vi "APC_PC_UI_System.vi"() -> ()   [LabVIEW 2020]
uses:
  controls/APC_PIDcontrolSettings.ctl
  <vilib>/Modbus/master/Create Master Instance (TCP).vi
  <vilib>/Modbus/master/Modbus Master.lvclass
panel:
  in  "Tab Control 2":enum32{"System view", "MTR interface", "Other"}(tab)
  out "WF-PT-012avg":dbl caption="bar" format="%#.2f"
  out "NG_CL_inner":bool
  in  "Ar_direct":bool
  in  "Ar_CL_inner":bool
  in  "AR-FT-001-REF":dbl caption="kg/h" format="%#.2f"
  in  "O2_direct":bool
  in  "Tcoolant_direct":bool
  in  "Toil_direct":bool
  in  "Texh_direct":bool
  out "SW-TT-009":dbl caption="ºC" format="%#.1f"
  out "NGDI-TT-001":dbl caption="ºC" format="%#.1f"
  out "NGDI-PT-001":dbl caption="bar" format="%#.2f"
  out "NG-TT-001":dbl caption="ºC" format="%#.1f"
  out "NG-PT-001":dbl caption="bar" format="%#.2f"
  in  "O2_FF_NG":bool
  out "Emergency shutdown":bool
  out "Pre-operation":bool
  out "Operation":bool
  out "Start":bool
  out "Idle":bool
  out "Shutdown":bool
  out "MTR errors":bool[](array[boolean])
  out "HB":bool
  out "Control from LV":bool
  in  "MTR_CO2out_CL":bool
  in  "IMEP-REF":dbl caption="l" format="%#.2f"
  out "NG_CL_outer_IMEP":bool caption="NG_CL_outer"
  out "NG_CL_outer_Nm":bool caption="NG_CL_outer"
  in  "TORQUE-REF":dbl caption="l" format="%#.2f"
  out "9056":bool
  out "9049":bool
  out "TORQUE":dbl caption="Nm" format="%#.2f"
  in  "Toil_CL_outer":bool
  out "Stand-by":bool
  out "Motoring":bool
  out "Firing":bool
  out "Idling":bool
  out "Emergency":bool
  in  "Tcoolant_CL":bool
  in  "Toil_CL_inner":bool
  out "Pmax-6":dbl caption="bar" format="%#.2f"
  out "Pmax-5":dbl caption="bar" format="%#.2f"
  out "Pmax-4":dbl caption="bar" format="%#.2f"
  out "Pmax-3":dbl caption="bar" format="%#.2f"
  out "Pmax-2":dbl caption="bar" format="%#.2f"
  out "Pmax-1":dbl caption="bar" format="%#.2f"
  out "IMEP-6":dbl caption="bar" format="%#.2f"
  out "IMEP-5":dbl caption="bar" format="%#.2f"
  out "IMEP-4":dbl caption="bar" format="%#.2f"
  out "IMEP-3":dbl caption="bar" format="%#.2f"
  out "IMEP-2":dbl caption="bar" format="%#.2f"
  out "IMEP-1":dbl caption="bar" format="%#.2f"
  out "PC-TT-006":dbl caption="ºC" format="%#.1f"
  out "PC-TT-005":dbl caption="ºC" format="%#.1f"
  out "PC-TT-004":dbl caption="ºC" format="%#.1f"
  out "PC-TT-003":dbl caption="ºC" format="%#.1f"
  out "PC-TT-002":dbl caption="ºC" format="%#.1f"
  out "PC-TT-001":dbl caption="ºC" format="%#.1f"
  out "EO-PT-001":dbl caption="bar" format="%#.2f"
  out "EO-TT-002":dbl caption="ºC" format="%#.1f"
  out "RPM":dbl caption="rpm" format="%#.1f"
  in  "EMERGENCY STOP":bool
  in  "Clear warning":bool
  in  "Exhaust vent":bool
  in  "Cross vent":bool
  in  "Intake vent":bool
  in  "O2":bool
  in  "Ar":bool
  in  "NG":bool
  in  "MTR_BackPressure_CL":bool
  in  "Texh_CL_outer":bool
  in  "Texh_CL_inner":bool
  in  "MTR_BackFlow_CL":bool
  in  "CO2_CL_inner":bool
  in  "CO2_CL_outer":bool
  out "NG_CL_outer_lambda":bool caption="NG_CL_outer"
  in  "O2_CL":bool
  in  "AR_CL_outer":bool
  out "AT201_CO2Conc":dbl caption="[% CO2]" format="%#.2f"
  in  "AIC201_CO2_ConcTarget":dbl caption="[% CO2]" format="%#.2f"
  in  "PV300_VlvPosTarget_pc":dbl caption="%" format="%#.2f"
  out "PV300_VlvPos_pc_fb":dbl caption="%" format="%#.2f"
  out "PT300_Pressure_kPa":dbl caption="bar" format="%#.2f"
  in  "PV300_PressTarget_kPa":dbl caption="bar" format="%#.2f"
  in  "WF-TT-004-REF":dbl caption="ºC"
  out "AT103_CO2Conc":dbl caption="[% CO2]" format="%#.2f"
  in  "AIC103_CO2_ConcTarget":dbl caption="[% CO2]" format="%#.2f"
  in  "PV103_VlvPosTarget_pc":dbl caption="%" format="%#.2f"
  out "PV103_VlvPos_pc_fb":dbl caption="%" format="%#.2f"
  out "PT103_Pressure_kPa":dbl caption="bar" format="%#.2f"
  in  "PV103_PressTarget_kPa":dbl caption="bar" format="%#.2f"
  in  "FV301_VlvPosTarget_pc":dbl caption="%" format="%#.2f"
  out "FV301_VlvPos_pc_fb":dbl caption="%" format="%#.2f"
  in  "FV301_FlowTarget_kgh":dbl caption="kg/h" format="%#.2f"
  in  "SW-FC-004-REF":dbl caption="%" format="%#.2f"
  out "SW-FC-004":dbl caption="%" format="%#.2f"
  in  "SW-FT-002-REF":dbl caption="kg/h" format="%#.2f"
  in  "SW-FC-008-REF":dbl caption="%" format="%#.2f"
  out "SW-FC-009":dbl caption="%" format="%#.2f"
  in  "EO-TT-001-REF":dbl caption="ºC"
  out "EO-TT-001":dbl caption="ºC" format="%#.1f"
  in  "SW-FT-004-REF":dbl caption="kg/h" format="%#.2f"
  out "WF-TT-007":dbl caption="ºC" format="%#.1f"
  out "WF-PT-016":dbl caption="bar" format="%#.2f"
  out "WF-PT-014":dbl caption="bar" format="%#.2f"
  out "WF-TT-003":dbl caption="ºC" format="%#.1f"
  in  "NG-FC-001-REF":dbl caption="kg/h" format="%#.2f"
  out "NG-FC-001":dbl caption="kg/h" format="%#.2f"
  out "ExhVent":bool
  out "O2":bool
  out "Ar":bool
  out "NG":bool
  out "CrossVent":bool
  out "IntVent":bool
  in  "EC-FC-001-REF":dbl caption="%"
  out "EC-FC-001":dbl caption="%"
  in  "EC-TT-001-REF":dbl caption="ºC"
  in  "WF-OA-002-REF":dbl caption="l" format="%#.2f"
  in  "AR-PC-002-REF":dbl caption="bar" format="%#.2f"
  in  "O2-FC-001-REF":dbl caption="kg/h" format="%#.2f"
  in  "WF-OA-001-REF":dbl caption="[% O2]" format="%#.2f"
  out "WF-TT-004":dbl caption="ºC" format="%#.1f"
  out "PT104_Pressure_kPa":dbl caption="bar" format="%#.2f"
  out "PT106_Pressure_kPa":dbl caption="bar" format="%#.2f"
  out "C101_CompSpeed_rpm":dbl caption="rpm"
  out "SW-TT-002":dbl caption="ºC" format="%#.1f"
  out "SW-TT-001":dbl caption="ºC" format="%#.1f"
  out "SW-TT-003":dbl caption="ºC" format="%#.1f"
  out "SW-TT-004":dbl caption="ºC" format="%#.1f"
  out "SW-TT-008":dbl caption="ºC" format="%#.1f"
  out "SW-TT-007":dbl caption="ºC" format="%#.1f"
  out "SW-TT-005":dbl caption="ºC" format="%#.1f"
  out "SW-TT-006":dbl caption="ºC" format="%#.1f"
  out "EC-TT-001":dbl caption="ºC" format="%#.1f"
  out "EC-TT-002":dbl caption="ºC" format="%#.1f"
  out "WF-OA-001":dbl caption="[% O2]" format="%#.2f"
  out "WF-PT-005avg":dbl caption="bar" format="%#.2f"
  out "WF-PT-004":dbl caption="bar" format="%#.2f"
  out "WF-OA-002":dbl caption="l" format="%#.2f"
  out "WF-TT-002":dbl caption="ºC" format="%#.1f"
  out "O2-TT-001":dbl caption="ºC" format="%#.1f"
  out "O2-PT-001":dbl caption="bar" format="%#.2f"
  out "AR-TT-001":dbl caption="ºC" format="%#.1f"
  out "AR-PT-001":dbl caption="bar" format="%#.2f"
  out "WF-TT-001":dbl caption="ºC" format="%#.1f"
  out "WF-PT-001":dbl caption="bar" format="%#.2f"
  out "FT301_Flow_kgh":dbl caption="kg/h" format="%#.2f"
  out "SW-FT-002":dbl caption="kg/h" format="%#.2f"
  out "SW-FT-003":dbl caption="kg/h" format="%#.2f"
  out "SW-FT-001":dbl caption="kg/h" format="%#.2f"
  out "SW-FT-004":dbl caption="kg/h" format="%#.2f"
  out "O2-FC-001":dbl caption="kg/h" format="%#.2f"
  out "NG-FT-001":dbl caption="kg/h" format="%#.2f"
  out "AR-FT-001":dbl caption="kg/h" format="%#.2f"
  out "NGDI-FT-001":dbl caption="kg/h" format="%#.1f"
  in  "WF-PT-003-REF":dbl caption="bar" format="%#.2f"
  out "NOx":dbl caption="[ppm NOx]" format="%#.1f"
  in  "port (502)":u16=502
  in  "Slave address":string="172.22.11.1"
  out "error out":errorcluster
  in  "min 2":sgl[](array[numeric])=[0.0, 0.0, 0.0, 0.0, 0.0, 0.0, 0.0, 0.0, 0.0, 0.0, 0.0, 0.0, 0.0, 0.0, 0.0, 0.0, 0.0, 0.0, 0.0]
  in  "max 2":sgl[](array[numeric])=[100.0, 100.0, 300.0, 300.0, 100.0, 100.0, 100.0, 100.0, 500.0, 500.0, 100.0, 100.0, 200.0, 200.0, 100.0, 100.0, 40000.0, 300.0, 600.0]
  out "MTR modbus floats":sgl[](array[numeric])
  in  "max":sgl[](array[numeric])=[100.0, 300.0, 100.0, 100.0, 500.0, 100.0, 200.0, 100.0]
  in  "min":sgl[](array[numeric])=[0.0, 0.0, 0.0, 0.0, 0.0, 0.0, 0.0, 0.0]
  in  "Send2MTRuint16":u16[](array[numeric])=[0, 0, 0]
  in  "Send2MTRfloats":sgl[](array[numeric])=[0.0, 0.0, 0.0, 0.0, 0.0, 0.0, 0.0, 0.0]
  out "MTR modbus u16":u16[](array[numeric])
  out "Texh control mode":u8
  out "PV300_Ctrl_Mode":u16
  out "FV301_Ctrl_Mode":u16
  out "NG control mode":u8
  out "Ar control mode":u8
  out "O2 control mode":u8
  out "Tcoolant control  mode":u8
  out "PV103_Ctrl_Mode":u16
  out "OverrideFromMain":bool
  out "Toil control mode":u8
  # "monarch APC v0.1"
  # "NG"
  # "T exh"
  # "IMEP"
  # "peak P"
  # "AR"
  # "NG FF"
  # "coolant"
  # "O2"
  # "oil"
  # "RT HB"
  # "Main switches"
  # "Membrane warnings"
  # "0 - M101 inlet T HH\n1 - M101 inlet p HH\n2 - S101 level HH\n3 - C101 inlet p LL\n4 - C101 inlet p HH\n5 - C101 outlet p HH\n6 - C101 outlet T HH\n7 - Oil p LL\n8 - Oil T HH\n9 - S102 level HH\n10 - M102 inlet T HH\n11 - CO2 exhaust T LL"
  # "M101"
  # "S102"
  # "C101"
  # "S101"
  # "drain"
  # "Membrane state"
  # "CO2"
  # "M102"
  # "AIC103_CO2_ConcTarget\nPV103_PressTarget_kPa\nPV103_VlvPosTarget_pc\nAIC201_CO2_ConcTarget\nFV301_FlowTarget_kgh\nFV301_VlvPosTarget_pc\nPV300_PressTarget_kPa\nPV300_VlvPosTarget_pc"
  # "PV103_Ctrl_Mode\nFV301_Ctrl_Mode\nPV300_Ctrl_Mode"
  # "AIC103_CO2_ConcTarget_ack\nAT103_CO2Conc\nPV103_PressTarget_kPa_ack\nPT103_Pressure_kPa\nPV103_VlvPosTarget_pc_ack\nPV103_VlvPos_pc_fb\nAIC201_CO2_ConcTarget_ack\nAT201_CO2Conc\nFV301_FlowTarget_kgh_ack\nFT301_Flow_kgh\nFV301_VlvPosTarget_pc_ack\nFV301_VlvPos_pc_fb\nPV300_PressTarget_kPa_ack\nPT300_Pressure_kPa\nPV300_VlvPosTarget_pc_ack\nPV300_VlvPos_pc_fb\nC101_CompSpeed_rpm\nPT104_Pressure_kPa\nPT106_Pressure_kPa"
  # "PLC_Manual_Control\nMTR_State\nMTR_HeartBeat\nPV103_Ctrl_Mode_act\nFV301_Ctrl_Mode_act\nPV300_Ctrl_Mode_act\nMTR_Diagnostic_Status"
  # "0 - Undefined\n1 - Idle\n2 - Start\n3 - Pre-Operation\n4 - Operation\n5 - ShutDown\n6 - Emergency ShutDown (ESD triggered!)"
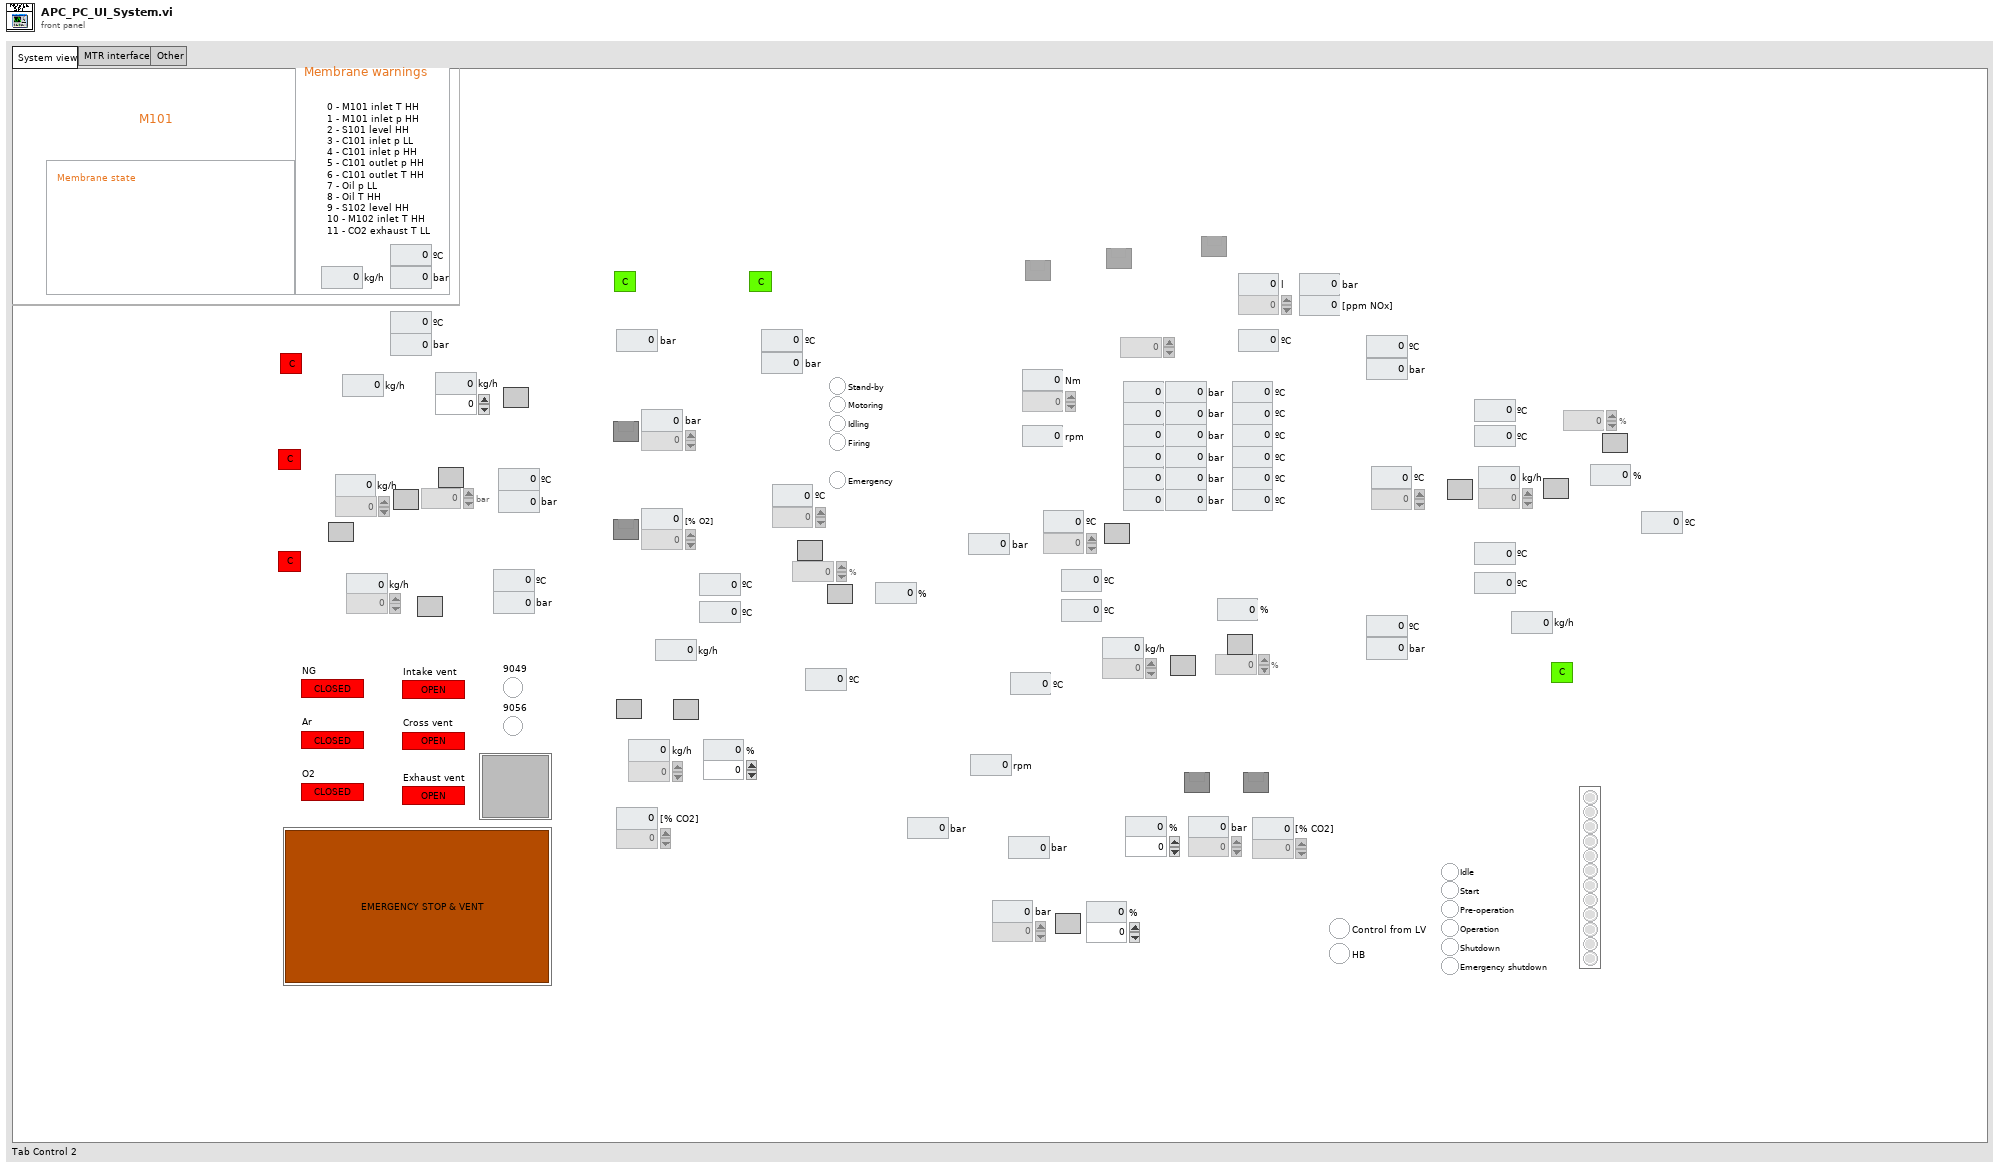
[diagram p1: front panel]
types:
  T1 = typedef "APC_PIDcontrolSettings.ctl" = cluster{"NG":bool, "Ar":bool, "O2":bool, "Intake vent":bool, "Cross vent":bool, "Exhaust vent":bool, "NG control mode":u8, "NG-FC-001-REF":dbl, "WF-OA-002-REF":dbl, "IMEP-REF":dbl, "Nm-REF":dbl, "Ar control mode":u8, "AR-PC-002-REF":dbl, "WF-PT-004-REF":dbl, "O2 control mode":u8, "O2-FC-001-REF":dbl, "WF-OA-001-REF":dbl, "Tcoolant control  mode":u8, "EC-FC-001-REF":dbl, "EC-TT-001-REF":dbl, "Texh control mode":u8, "SW-FC-004-REF":dbl, "SW-FT-002-REF":dbl, "WF-TT-004-REF":dbl, "Toil control mode":u8, "SW-FC-009-REF":dbl, "SW-FT-004-REF":dbl, "EO-TT-001-REF":dbl, "AIC201_CO2_ConcTarget":dbl, "O2_FF_NG":bool, "Dyno control mode":u8, "Membrane control mode":u8, "AR-FT-001-REF":dbl, "MTR modbus floats":sgl[], "MTR modbus u16":u16[], "MTR HB":bool, "PC_HB":bool, "EMERGENCY STOP":bool}
  T2 = enum8{"Enabled", "Disabled", "Disabled and Grayed Out"}
  T3 = typedef "APC_VisualizationCluster_v2.ctl" = cluster{"AR-FT-001":dbl, "AR-PT-001":dbl, "AR-TT-001":dbl, "AT103_CO2Conc":dbl, "AT201_CO2Conc":dbl, "C101_CompSpeed_rpm":dbl, "CO2 [%]":dbl, "EC-FC-001":dbl, "EC-TT-001":dbl, "EC-TT-002":dbl, "PC-TT-001":dbl, "PC-TT-002":dbl, "PC-TT-003":dbl, "PC-TT-004":dbl, "PC-TT-005":dbl, "PC-TT-006":dbl, "EO-PT-001":dbl, "EO-TT-001":dbl, "EO-TT-002":dbl, "FT301_Flow_kgh":dbl, "FV301_VlvPos_pc_fb":dbl, "IMEPn1":dbl, "IMEPn2":dbl, "IMEPn3":dbl, "IMEPn4":dbl, "IMEPn5":dbl, "IMEPn6":dbl, "IMEPstd1":dbl, "IMEPstd2":dbl, "IMEPstd3":dbl, "IMEPstd4":dbl, "IMEPstd5":dbl, "IMEPstd6":dbl, "NG-FC-001":dbl, "NG-FT-001":dbl, "NG-PT-001":dbl, "NG-TT-001":dbl, "NGDI-FT-001":dbl, "NGDI-PT-001":dbl, "NGDI-TT-001":dbl, "WF-OA-002-NOx":dbl, "TORQUE":dbl, "WF-OA-002-O2corr":dbl, "O2-FC-001":dbl, "O2-PT-001":dbl, "O2-TT-001":dbl, "PT103_Pressure_kPa":dbl, "PT104_Pressure_kPa":dbl, "PT106_Pressure_kPa":dbl, "PT300_Pressure_kPa":dbl, "PV103_VlvPos_pc_fb":dbl, "PV300_VlvPos_pc_fb":dbl, "MaxPcyl1":dbl, "MaxPcyl2":dbl, "MaxPcyl3":dbl, "MaxPcyl4":dbl, "MaxPcyl5":dbl, "MaxPcyl6":dbl, "SW-FC-004":dbl, "SW-FC-009":dbl, "SW-FT-001":dbl, "SW-FT-002":dbl, "SW-FT-003":dbl, "SW-FT-004":dbl, "SW-TT-001":dbl, "SW-TT-002":dbl, "SW-TT-003":dbl, "SW-TT-004":dbl, "SW-TT-005":dbl, "SW-TT-006":dbl, "SW-TT-007":dbl, "SW-TT-008":dbl, "WF-OA-001":dbl, "WF-OA-002":dbl, "WF-PT-001":dbl, "WF-PT-004":dbl, "WF-PT-005avg":dbl, "WF-PT-014":dbl, "WF-PT-015":dbl, "WF-PT-016":dbl, "WF-TT-001":dbl, "WF-TT-002":dbl, "WF-TT-003":dbl, "WF-TT-004":dbl, "WF-TT-007":dbl, "EngineSpeed_rpm":dbl, "SystemState":dbl, "CylPresWarnings":dbl, "CylPresErrors":dbl, "MAPO1":dbl, "MAPO2":dbl, "MAPO3":dbl, "MAPO4":dbl, "MAPO5":dbl, "MAPO6":dbl, "CA50_1":dbl, "CA50_2":dbl, "CA50_3":dbl, "CA50_4":dbl, "CA50_5":dbl, "CA50_6":dbl, "SparkTiming":dbl, "SW-TT-009":dbl, "NG-FV-001":dbl, "O2-PV-004":dbl, "AR-PV-004":dbl, "WF-FC-001":dbl, "WF-FC-002":dbl, "WF-FC-003":dbl, "WF-PT-012avg":dbl}
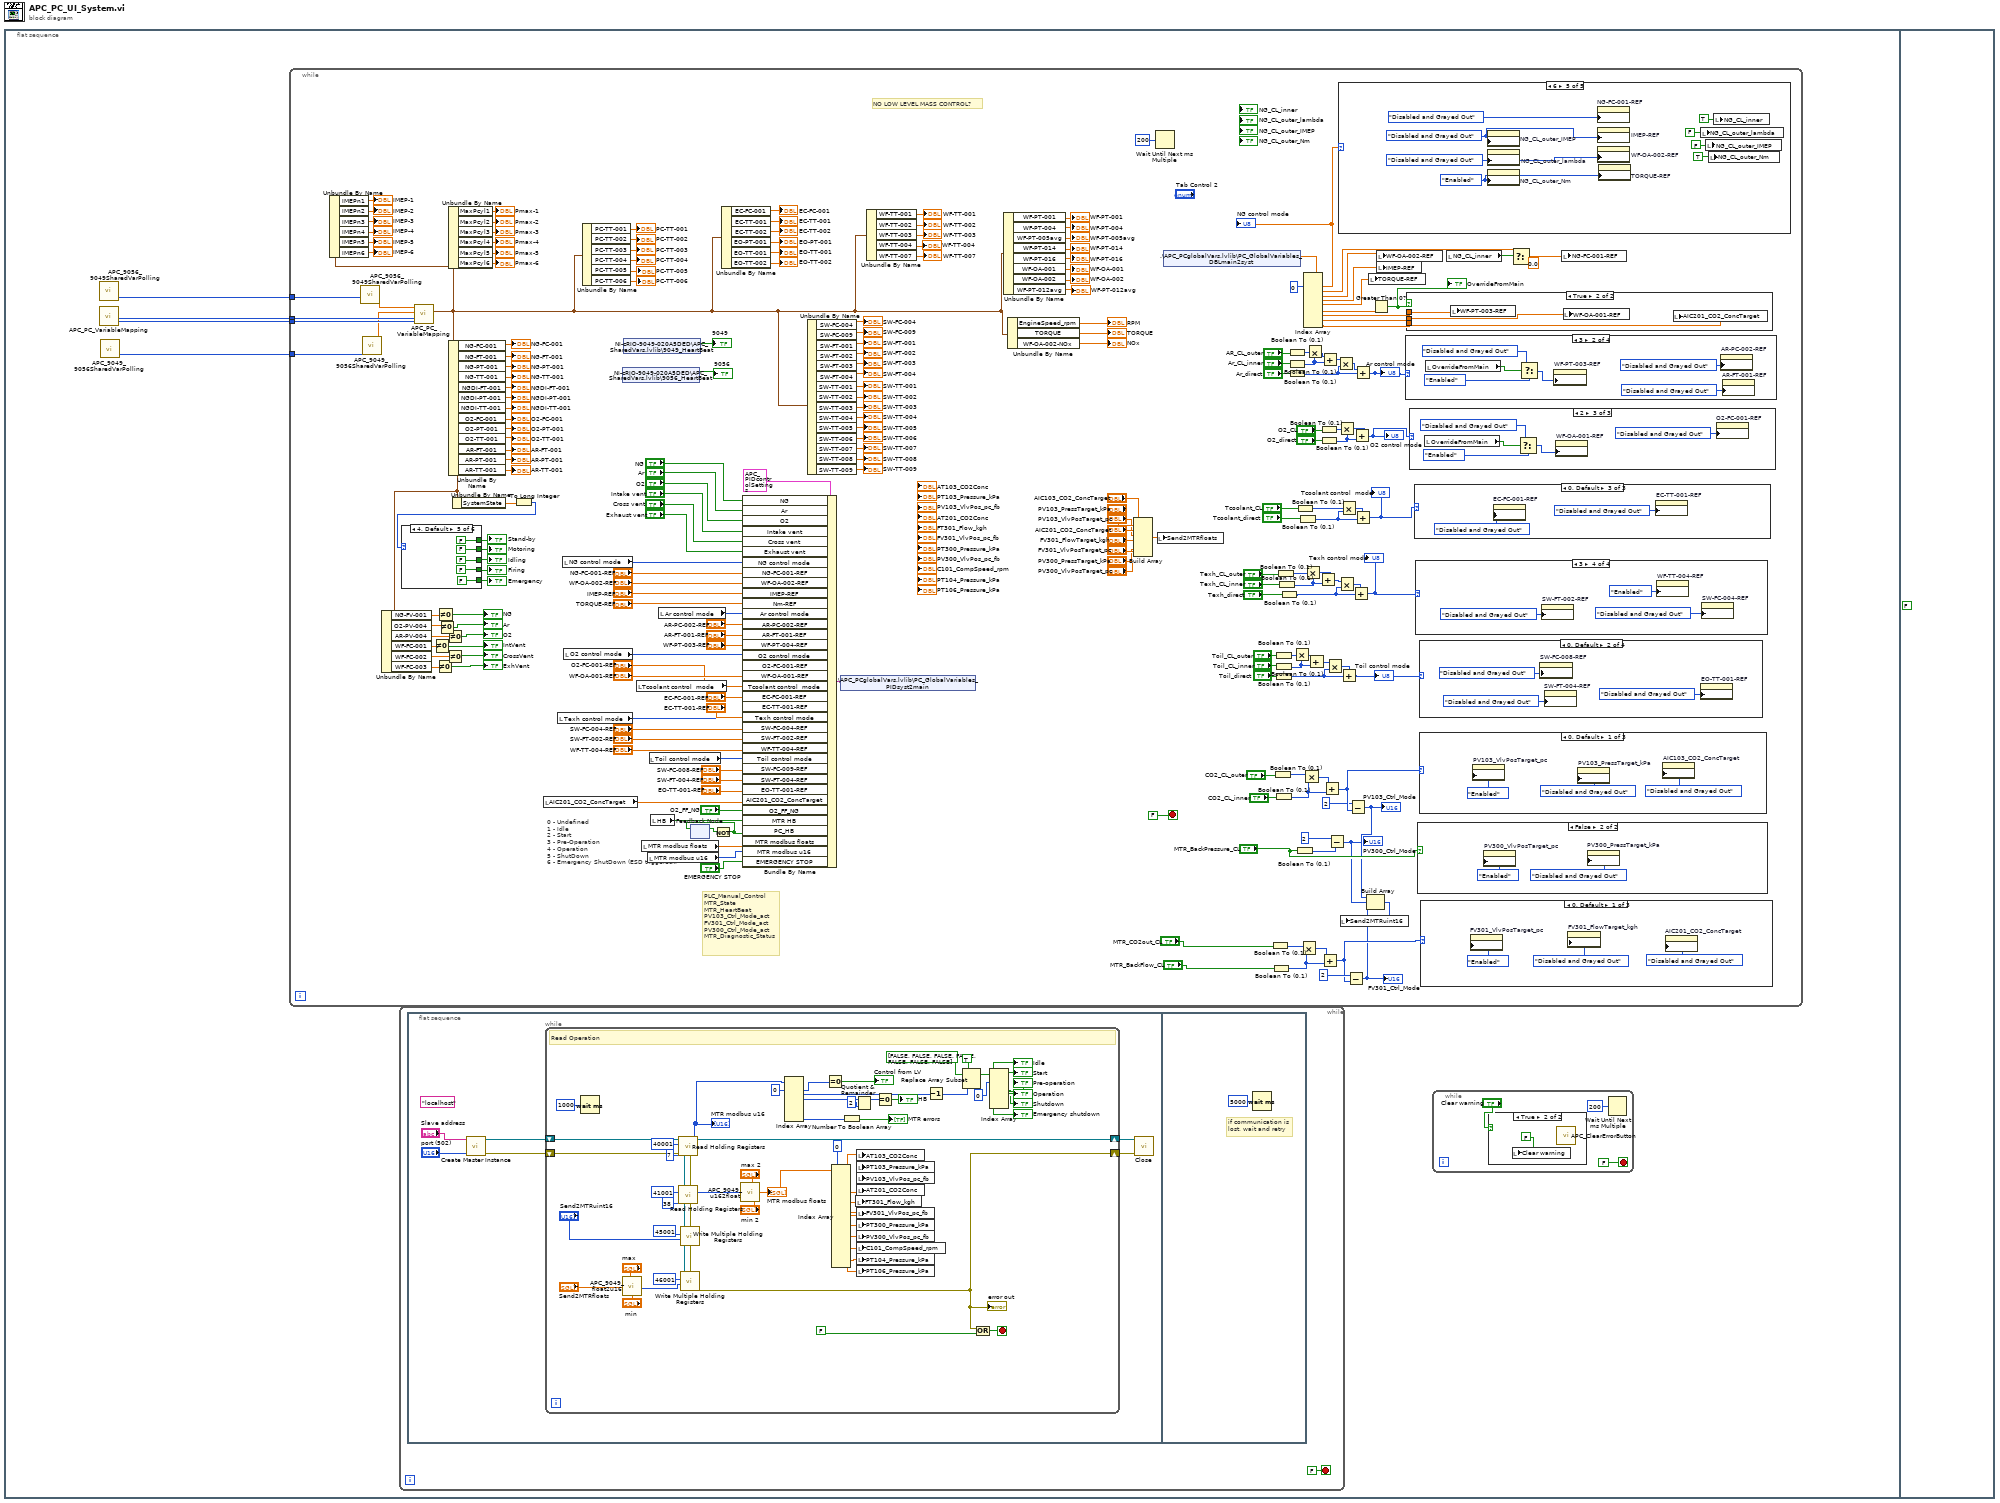
[diagram p0: block diagram]
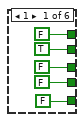
[diagram p3: hidden frame]
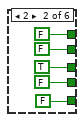
[diagram p4: hidden frame]
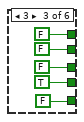
[diagram p5: hidden frame]
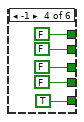
[diagram p6: hidden frame]
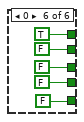
[diagram p7: hidden frame]
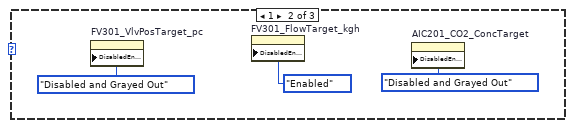
[diagram p9: hidden frame]
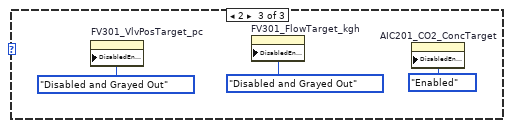
[diagram p10: hidden frame]
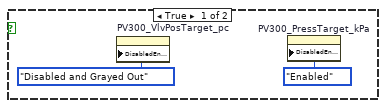
[diagram p11: hidden frame]
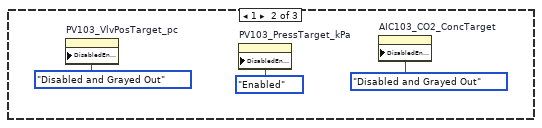
[diagram p12: hidden frame]
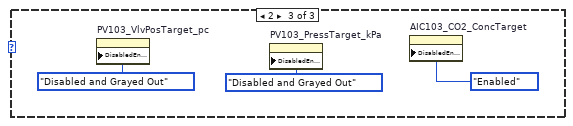
[diagram p13: hidden frame]
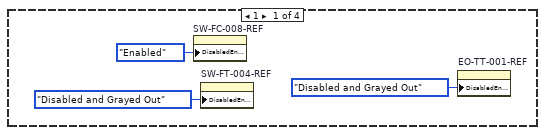
[diagram p14: hidden frame]
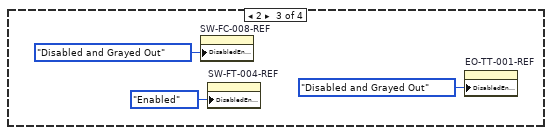
[diagram p15: hidden frame]
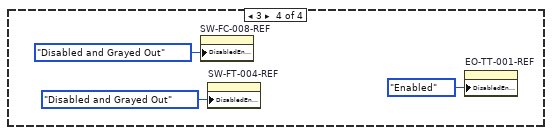
[diagram p16: hidden frame]
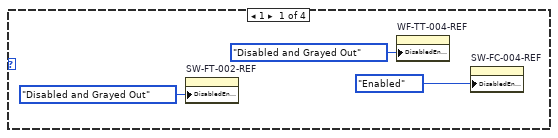
[diagram p17: hidden frame]
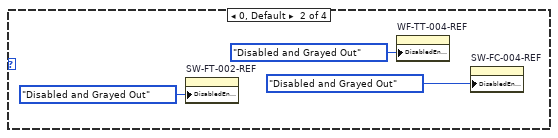
[diagram p18: hidden frame]
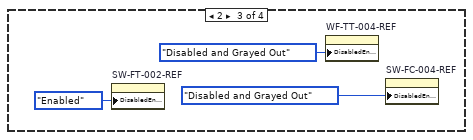
[diagram p19: hidden frame]
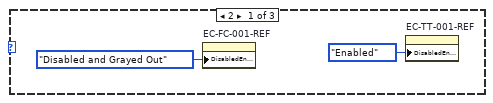
[diagram p20: hidden frame]
diagram:
  n1 = flat-sequence {
    frame #0 {
      n2 = call "APC_9056_9049SharedVarPolling.vi"() -> ("Number of signals (out)"=w2:i32)  [unwired: 1 in, 1 out]
      n3 = call "APC_PC_VariableMapping.vi"() -> ("Index 9056"=w3:i32[], "Index 9049"=w4:i32[])  [unwired: 4 in, 1 out]
      n4 = call "APC_9049_9056SharedVarPolling.vi"() -> ("Number of signals (out)"=w1:i32)  [unwired: 1 in, 3 out]
      n5 = while {
        tunnel: w4 -> [w298]
        tunnel: w3 -> [w297]
        tunnel: w2 -> [w296]
        tunnel: w1 -> [w295]
        stop <- FALSE stop-if-true
        # "0 - Undefined\n1 - Idle\n2 - Start\n3 - Pre-Operation\n4 - Operation\n5 - ShutDown\n6 - Emergency ShutDown (ESD triggered!)"
        # "PLC_Manual_Control\nMTR_State\nMTR_HeartBeat\nPV103_Ctrl_Mode_act\nFV301_Ctrl_Mode_act\nPV300_Ctrl_Mode_act\nMTR_Diagnostic_Status"
        # "NO LOW LEVEL MASS CONTROL?"
        n6 = call "APC_9056_9049SharedVarPolling.vi"("Number of signals"=w296) -> ("9049_CycleAveragedVariables"=w293:dbl[])  [unwired: 1 out]
        n7 = call "APC_9049_9056SharedVarPolling.vi"("Number of signals"=w295) -> ("9056 IO"=w292:dbl[])  [unwired: 3 out]
        n8 = call "APC_PC_VariableMapping.vi"("Index of array for 9056"=w297, "Index of array for 9049"=w298, "9056 IO"=w292, "9049_CycleAveragedVariables"=w293) -> ("Output cluster"=w96:T3)  [unwired: 2 out]
        n9 = Unbundle By Name(w96) -> ("IMEPn1"=→"IMEP-1":dbl, "IMEPn2"=→"IMEP-2":dbl, "IMEPn3"=→"IMEP-3":dbl, "IMEPn4"=→"IMEP-4":dbl, "IMEPn5"=→"IMEP-5":dbl, "IMEPn6"=→"IMEP-6":dbl)
        n10 = Unbundle By Name(w96) -> ("NG-FV-001"=w95:dbl, "O2-PV-004"=w93:dbl, "AR-PV-004"=w91:dbl, "WF-FC-001"=w89:dbl, "WF-FC-002"=w87:dbl, "WF-FC-003"=w85:dbl)
        n11 = Not Equal To 0?(x=w89) -> (x != 0?=→"IntVent":bool)
        n12 = Not Equal To 0?(x=w85) -> (x != 0?=→"ExhVent":bool)
        n13 = Not Equal To 0?(x=w95) -> (x != 0?=→"NG":bool)
        n14 = Not Equal To 0?(x=w93) -> (x != 0?=→"Ar":bool)
        n15 = Not Equal To 0?(x=w91) -> (x != 0?=→"O2":bool)
        n16 = Not Equal To 0?(x=w87) -> (x != 0?=→"CrossVent":bool)
        n17 = Unbundle By Name(w96) -> ("MaxPcyl1"=→"Pmax-1":dbl, "MaxPcyl2"=→"Pmax-2":dbl, "MaxPcyl3"=→"Pmax-3":dbl, "MaxPcyl4"=→"Pmax-4":dbl, "MaxPcyl5"=→"Pmax-5":dbl, "MaxPcyl6"=→"Pmax-6":dbl)
        n18 = Unbundle By Name(w96) -> ("NG-FC-001"=→"NG-FC-001":dbl, "NG-FT-001"=→"NG-FT-001":dbl, "NG-PT-001"=→"NG-PT-001":dbl, "NG-TT-001"=→"NG-TT-001":dbl, "NGDI-FT-001"=→"NGDI-FT-001":dbl, "NGDI-PT-001"=→"NGDI-PT-001":dbl, "NGDI-TT-001"=→"NGDI-TT-001":dbl, "O2-FC-001"=→"O2-FC-001":dbl, "O2-PT-001"=→"O2-PT-001":dbl, "O2-TT-001"=→"O2-TT-001":dbl, "AR-FT-001"=→"AR-FT-001":dbl, "AR-PT-001"=→"AR-PT-001":dbl, "AR-TT-001"=→"AR-TT-001":dbl)
        n19 = Unbundle By Name(w96) -> ("SystemState"=w182:dbl)
        n20 = To Long Integer(number=w182) -> (32bit integer=w102:i32)
        n21 = case shown="4, Default" w102 {
          tunnel: [FALSE ("Stand-by") FALSE ("Stand-by") FALSE ("Stand-by") FALSE ("Stand-by") FALSE ("Stand-by") TRUE ("Stand-by")] -> w101
          tunnel: [TRUE ("Stand-by") FALSE ("Stand-by") FALSE ("Stand-by") FALSE ("Stand-by") FALSE ("Stand-by") FALSE ("Stand-by")] -> w100
          tunnel: [FALSE ("Stand-by") FALSE ("Stand-by") FALSE ("Stand-by") TRUE ("Stand-by") FALSE ("Stand-by") FALSE ("Stand-by")] -> w97
          tunnel: [FALSE ("Stand-by") TRUE ("Stand-by") FALSE ("Stand-by") FALSE ("Stand-by") FALSE ("Stand-by") FALSE ("Stand-by")] -> w99
          tunnel: [FALSE ("Stand-by") FALSE ("Stand-by") TRUE ("Stand-by") FALSE ("Stand-by") FALSE ("Stand-by") FALSE ("Stand-by")] -> w98
          frame 1 {
          }
          frame 2 {
          }
          frame 3 {
          }
          frame -1 {
          }
          frame 4, Default {
          }
          frame 0 {
          }
        }
        "Emergency" <- w97
        "Idling" <- w99
        "Firing" <- w98
        "Motoring" <- w100
        "Stand-by" <- w101
        n22 = local read "AIC201_CO2_ConcTarget"() -> (w150:dbl)
        n23 = local read "Texh control mode"() -> (w190:u8)
        n24 = local read "NG control mode"() -> (w204:u8)
        n25 = local read "O2 control mode"() -> (w194:u8)
        n26 = Unbundle By Name(w96) -> ("PC-TT-001"=→"PC-TT-001":dbl, "PC-TT-002"=→"PC-TT-002":dbl, "PC-TT-003"=→"PC-TT-003":dbl, "PC-TT-004"=→"PC-TT-004":dbl, "PC-TT-005"=→"PC-TT-005":dbl, "PC-TT-006"=→"PC-TT-006":dbl)
        n27 = shared-variable "NI-cRIO-9049-020A5DED\\APC_SharedVars.lvlib\\9056_HeartBeat"() -> (→"9056":bool)  [unwired: 1 in, 1 out]
        n28 = shared-variable "NI-cRIO-9049-020A5DED\\APC_SharedVars.lvlib\\9049_HeartBeat"() -> (→"9049":bool)  [unwired: 1 in, 1 out]
        n29 = local read "Tcoolant control  mode"() -> (w192:u8)
        n30 = local read "MTR modbus floats"() -> (w79:sgl[])
        n31 = local read "MTR modbus u16"() -> (w80:u16[])
        n32 = local read "Toil control mode"() -> (w186:u8)
        n33 = local read "HB"() -> (w81:bool)
        n34 = local read "Ar control mode"() -> (w198:u8)
        n35 = feedback #1() -> (w77:bool)  [unwired: 1 in]
        n36 = Not(x=w77) -> (.not. x?=w78:bool)
        n37 = feedback-in #1(w78) -> ()
        n38 = Unbundle By Name(w96) -> ("EC-FC-001"=→"EC-FC-001":dbl, "EC-TT-001"=→"EC-TT-001":dbl, "EC-TT-002"=→"EC-TT-002":dbl, "EO-PT-001"=→"EO-PT-001":dbl, "EO-TT-001"=→"EO-TT-001":dbl, "EO-TT-002"=→"EO-TT-002":dbl)
        n39 = Bundle By Name(cluster=T1 {"NG"=FALSE, "Ar"=FALSE, "O2"=FALSE, "Intake vent"=FALSE, "Cross vent"=FALSE, "Exhaust vent"=FALSE, "NG control mode"=0, "NG-FC-001-REF"=0.0, "WF-OA-002-REF"=0.0, "IMEP-REF"=0.0, "Nm-REF"=0.0, "Ar control mode"=0, "AR-PC-002-REF"=0.0, "WF-PT-004-REF"=0.0, "O2 control mode"=0, "O2-FC-001-REF"=0.0, "WF-OA-001-REF"=0.0, "Tcoolant control  mode"=0, "EC-FC-001-REF"=0.0, "EC-TT-001-REF"=0.0, "Texh control mode"=0, "SW-FC-004-REF"=0.0, "SW-FT-002-REF"=0.0, "WF-TT-004-REF"=0.0, "Toil control mode"=0, "SW-FC-009-REF"=0.0, "SW-FT-004-REF"=0.0, "EO-TT-001-REF"=0.0, "AIC201_CO2_ConcTarget"=0.0, "O2_FF_NG"=FALSE, "Dyno control mode"=0, "Membrane control mode"=0, "AR-FT-001-REF"=0.0, "MTR modbus floats"=[0.0, 0.0, 0.0, 0.0, 0.0, 0.0, 0.0, 0.0, 0.0, 0.0, 0.0, 0.0, 0.0, 0.0, 0.0, 0.0, 0.0, 0.0, 0.0], "MTR modbus u16"=[0, 0, 0, 0, 0, 0, 0], "MTR HB"=FALSE, "PC_HB"=FALSE, "EMERGENCY STOP"=FALSE} ("PID control references"), "NG"="NG", "Ar"="Ar", "O2"="O2", "Intake vent"="Intake vent", "Cross vent"="Cross vent", "Exhaust vent"="Exhaust vent", "NG control mode"=w204, "NG-FC-001-REF"="NG-FC-001-REF", "WF-OA-002-REF"="WF-OA-002-REF", "IMEP-REF"="IMEP-REF", "Nm-REF"="TORQUE-REF", "Ar control mode"=w198, "AR-PC-002-REF"="AR-PC-002-REF", "AR-FT-001-REF"="AR-FT-001-REF", "WF-PT-004-REF"="WF-PT-003-REF", "O2 control mode"=w194, "O2-FC-001-REF"="O2-FC-001-REF", "WF-OA-001-REF"="WF-OA-001-REF", "Tcoolant control  mode"=w192, "EC-FC-001-REF"="EC-FC-001-REF", "EC-TT-001-REF"="EC-TT-001-REF", "Texh control mode"=w190, "SW-FC-004-REF"="SW-FC-004-REF", "SW-FT-002-REF"="SW-FT-002-REF", "WF-TT-004-REF"="WF-TT-004-REF", "Toil control mode"=w186, "SW-FC-009-REF"="SW-FC-008-REF", "SW-FT-004-REF"="SW-FT-004-REF", "EO-TT-001-REF"="EO-TT-001-REF", "AIC201_CO2_ConcTarget"=w150, "O2_FF_NG"="O2_FF_NG", "MTR HB"=w81, "PC_HB"=w78, "MTR modbus floats"=w79, "MTR modbus u16"=w80, "EMERGENCY STOP"="EMERGENCY STOP") -> (w183:T1)
        n40 = Unbundle By Name(w96) -> ("SW-FC-004"=→"SW-FC-004":dbl, "SW-FC-009"=→"SW-FC-009":dbl, "SW-FT-001"=→"SW-FT-001":dbl, "SW-FT-002"=→"SW-FT-002":dbl, "SW-FT-003"=→"SW-FT-003":dbl, "SW-FT-004"=→"SW-FT-004":dbl, "SW-TT-001"=→"SW-TT-001":dbl, "SW-TT-002"=→"SW-TT-002":dbl, "SW-TT-003"=→"SW-TT-003":dbl, "SW-TT-004"=→"SW-TT-004":dbl, "SW-TT-005"=→"SW-TT-005":dbl, "SW-TT-006"=→"SW-TT-006":dbl, "SW-TT-007"=→"SW-TT-007":dbl, "SW-TT-008"=→"SW-TT-008":dbl, "SW-TT-009"=→"SW-TT-009":dbl)
        n41 = shared-variable ".\\APC_PCglobalVars.lvlib\\PC_GlobalVariables_PIDsyst2main"(w183) -> ()  [unwired: 1 in, 1 out]
        n42 = Unbundle By Name(w96) -> ("WF-TT-001"=→"WF-TT-001":dbl, "WF-TT-002"=→"WF-TT-002":dbl, "WF-TT-003"=→"WF-TT-003":dbl, "WF-TT-004"=→"WF-TT-004":dbl, "WF-TT-007"=→"WF-TT-007":dbl)
        n43 = Unbundle By Name(w96) -> ("WF-PT-001"=→"WF-PT-001":dbl, "WF-PT-004"=→"WF-PT-004":dbl, "WF-PT-005avg"=→"WF-PT-005avg":dbl, "WF-PT-014"=→"WF-PT-014":dbl, "WF-PT-016"=→"WF-PT-016":dbl, "WF-OA-001"=→"WF-OA-001":dbl, "WF-OA-002"=→"WF-OA-002":dbl, "WF-PT-012avg"=→"WF-PT-012avg":dbl)
        n44 = Unbundle By Name(w96) -> ("EngineSpeed_rpm"=→"RPM":dbl, "TORQUE"=→"TORQUE":dbl, "WF-OA-002-NOx"=→"NOx":dbl)
        n45 = Build Array("AIC103_CO2_ConcTarget", "PV103_PressTarget_kPa", "PV103_VlvPosTarget_pc", "AIC201_CO2_ConcTarget", "FV301_FlowTarget_kgh", "FV301_VlvPosTarget_pc", "PV300_PressTarget_kPa", "PV300_VlvPosTarget_pc") -> (w174:dbl[])
        n46 = Wait Until Next ms Multiple(millisecond multiple=u32 200) -> ()  [unwired: 1 out]
        n47 = local write "Send2MTRfloats"(w174) -> ()
        n48 = shared-variable ".\\APC_PCglobalVars.lvlib\\PC_GlobalVariables_DBLmain2syst"() -> (w221:dbl[])  [unwired: 1 in, 1 out]
        n49 = Boolean To (0,1)(Boolean="MTR_CO2out_CL") -> (0, 1=w163:i16)
        n50 = Boolean To (0,1)(Boolean="MTR_BackFlow_CL") -> (0, 1=w162:i16)
        n51 = Boolean To (0,1)(Boolean="CO2_CL_outer") -> (0, 1=w170:i16)
        n52 = Boolean To (0,1)(Boolean="Toil_CL_outer") -> (0, 1=w135:i16)
        n53 = Boolean To (0,1)(Boolean="Toil_CL_inner") -> (0, 1=w133:i16)
        n54 = Boolean To (0,1)(Boolean="Toil_direct") -> (0, 1=w131:i16)
        n55 = Boolean To (0,1)(Boolean="CO2_CL_inner") -> (0, 1=w169:i16)
        n56 = Boolean To (0,1)(Boolean="Texh_CL_outer") -> (0, 1=w220:i16)
        n57 = Boolean To (0,1)(Boolean="Texh_CL_inner") -> (0, 1=w218:i16)
        n58 = Boolean To (0,1)(Boolean="Texh_direct") -> (0, 1=w138:i16)
        n59 = Boolean To (0,1)(Boolean="AR_CL_outer") -> (0, 1=w112:i16)
        n60 = Boolean To (0,1)(Boolean="Ar_CL_inner") -> (0, 1=w110:i16)
        n61 = Boolean To (0,1)(Boolean="Ar_direct") -> (0, 1=w108:i16)
        n62 = Multiply(x=w135, y=w133) -> (x*y=w134:i16)
        n63 = Boolean To (0,1)(Boolean="MTR_BackPressure_CL") -> (0, 1=w165:i16)
        n64 = Boolean To (0,1)(Boolean="Tcoolant_CL") -> (0, 1=w122:i16)
        n65 = Boolean To (0,1)(Boolean="Tcoolant_direct") -> (0, 1=w123:i16)
        n66 = Multiply(x=w163, y=w162) -> (x*y=w164:i16)
        n67 = Multiply(x=w170, y=w169) -> (x*y=w171:i16)
        n68 = Index Array(array=w221, index #1=0 ("index")) -> (element #1=w226:dbl, element #2=w215:dbl, element #3=w225:dbl, element #4=w224:dbl, element #5=w223:dbl, element #6=w149:dbl, element #7=w147:dbl, element #8=w146:dbl, element #9=w145:dbl)  [unwired: 8 in]
        "NG control mode" <- w226
        n69 = Multiply(x=w220, y=w218) -> (x*y=w219:i16)
        n70 = Multiply(x=w112, y=w110) -> (x*y=w111:i16)
        n71 = Add(x=w134, y=w133) -> (x+y=w130:i16)
        n72 = Add(x=w219, y=w218) -> (x+y=w137:i16)
        n73 = Boolean To (0,1)(Boolean="O2_CL") -> (0, 1=w119:i16)
        n74 = Boolean To (0,1)(Boolean="O2_direct") -> (0, 1=w117:i16)
        n75 = Add(x=w111, y=w110) -> (x+y=w107:i16)
        n76 = Add(x=w164, y=w162) -> (x+y=w159:i16)
        n77 = Add(x=w171, y=w169) -> (x+y=w168:i16)
        n78 = Multiply(x=w130, y=w131) -> (x*y=w132:i16)
        n79 = Subtract(x=i16 2, y=w165) -> (x-y=w155:i16)
        "PV300_Ctrl_Mode" <- w155
        n80 = Multiply(x=w107, y=w108) -> (x*y=w109:i16)
        n81 = Multiply(x=w137, y=w138) -> (x*y=w139:i16)
        n82 = Multiply(x=w119, y=w117) -> (x*y=w118:i16)
        n83 = case shown="6" w226 {
          frame 0, Default {
            w411 = T2."Disabled and Grayed Out" ("Disabled")
            w410 = T2."Disabled and Grayed Out" ("Disabled")
            w409 = T2."Disabled and Grayed Out" ("Disabled")
            n84 = property on="NG_CL_outer_IMEP" class="Bool"("DisabledEnum"=w409) -> ()  [unwired: 2 in, 2 out]
            n85 = property on="NG_CL_outer_Nm" class="Bool"("DisabledEnum"=w411) -> ()  [unwired: 2 in, 2 out]
            n86 = property on="NG_CL_outer_lambda" class="Bool"("DisabledEnum"=w410) -> ()  [unwired: 2 in, 2 out]
            n87 = property on="NG-FC-001-REF" class="DigNum (strict)"("DisabledEnum"=T2."Disabled and Grayed Out" ("Disabled")) -> ()  [unwired: 2 in, 2 out]
            n88 = property on="IMEP-REF" class="DigNum (strict)"("DisabledEnum"=w409) -> ()  [unwired: 2 in, 2 out]
            n89 = property on="WF-OA-002-REF" class="DigNum (strict)"("DisabledEnum"=w410) -> ()  [unwired: 2 in, 2 out]
            n90 = property on="TORQUE-REF" class="DigNum (strict)"("DisabledEnum"=w411) -> ()  [unwired: 2 in, 2 out]
            n91 = local write "NG_CL_outer_lambda"(FALSE ("NG_CL_outer_lambda")) -> ()
            n92 = local write "NG_CL_outer_IMEP"(FALSE ("NG_CL_outer_IMEP")) -> ()
            n93 = local write "NG_CL_outer_Nm"(FALSE ("NG_CL_outer_Nm")) -> ()
            n94 = local write "NG_CL_inner"(FALSE ("NG_CL_inner")) -> ()
          }
          frame 1 {
            w419 = T2."Disabled and Grayed Out" ("Disabled")
            w418 = T2."Disabled and Grayed Out" ("Disabled")
            w417 = T2."Disabled and Grayed Out" ("Disabled")
            n95 = property on="NG_CL_outer_IMEP" class="Bool"("DisabledEnum"=w417) -> ()  [unwired: 2 in, 2 out]
            n96 = property on="NG_CL_outer_Nm" class="Bool"("DisabledEnum"=w419) -> ()  [unwired: 2 in, 2 out]
            n97 = property on="NG_CL_outer_lambda" class="Bool"("DisabledEnum"=w418) -> ()  [unwired: 2 in, 2 out]
            n98 = property on="NG-FC-001-REF" class="DigNum (strict)"("DisabledEnum"=T2."Enabled" ("Disabled")) -> ()  [unwired: 2 in, 2 out]
            n99 = property on="IMEP-REF" class="DigNum (strict)"("DisabledEnum"=w417) -> ()  [unwired: 2 in, 2 out]
            n100 = property on="WF-OA-002-REF" class="DigNum (strict)"("DisabledEnum"=w418) -> ()  [unwired: 2 in, 2 out]
            n101 = property on="TORQUE-REF" class="DigNum (strict)"("DisabledEnum"=w419) -> ()  [unwired: 2 in, 2 out]
            n102 = local write "NG_CL_outer_lambda"(FALSE ("NG_CL_outer_lambda")) -> ()
            n103 = local write "NG_CL_outer_IMEP"(FALSE ("NG_CL_outer_IMEP")) -> ()
            n104 = local write "NG_CL_outer_Nm"(FALSE ("NG_CL_outer_Nm")) -> ()
            n105 = local write "NG_CL_inner"(TRUE ("NG_CL_inner")) -> ()
          }
          frame 4 {
            w427 = T2."Disabled and Grayed Out" ("Disabled")
            w426 = T2."Enabled" ("Disabled")
            w425 = T2."Disabled and Grayed Out" ("Disabled")
            n106 = property on="NG_CL_outer_IMEP" class="Bool"("DisabledEnum"=w425) -> ()  [unwired: 2 in, 2 out]
            n107 = property on="NG_CL_outer_Nm" class="Bool"("DisabledEnum"=w427) -> ()  [unwired: 2 in, 2 out]
            n108 = property on="NG_CL_outer_lambda" class="Bool"("DisabledEnum"=w426) -> ()  [unwired: 2 in, 2 out]
            n109 = property on="NG-FC-001-REF" class="DigNum (strict)"("DisabledEnum"=T2."Disabled and Grayed Out" ("Disabled")) -> ()  [unwired: 2 in, 2 out]
            n110 = property on="IMEP-REF" class="DigNum (strict)"("DisabledEnum"=w425) -> ()  [unwired: 2 in, 2 out]
            n111 = property on="WF-OA-002-REF" class="DigNum (strict)"("DisabledEnum"=w426) -> ()  [unwired: 2 in, 2 out]
            n112 = property on="TORQUE-REF" class="DigNum (strict)"("DisabledEnum"=w427) -> ()  [unwired: 2 in, 2 out]
            n113 = local write "NG_CL_outer_lambda"(TRUE ("NG_CL_outer_lambda")) -> ()
            n114 = local write "NG_CL_outer_IMEP"(FALSE ("NG_CL_outer_IMEP")) -> ()
            n115 = local write "NG_CL_outer_Nm"(FALSE ("NG_CL_outer_Nm")) -> ()
            n116 = local write "NG_CL_inner"(TRUE ("NG_CL_inner")) -> ()
          }
          frame 5 {
            w435 = T2."Disabled and Grayed Out" ("Disabled")
            w434 = T2."Disabled and Grayed Out" ("Disabled")
            w433 = T2."Enabled" ("Disabled")
            n117 = property on="NG_CL_outer_IMEP" class="Bool"("DisabledEnum"=w433) -> ()  [unwired: 2 in, 2 out]
            n118 = property on="NG_CL_outer_Nm" class="Bool"("DisabledEnum"=w435) -> ()  [unwired: 2 in, 2 out]
            n119 = property on="NG_CL_outer_lambda" class="Bool"("DisabledEnum"=w434) -> ()  [unwired: 2 in, 2 out]
            n120 = property on="NG-FC-001-REF" class="DigNum (strict)"("DisabledEnum"=T2."Disabled and Grayed Out" ("Disabled")) -> ()  [unwired: 2 in, 2 out]
            n121 = property on="IMEP-REF" class="DigNum (strict)"("DisabledEnum"=w433) -> ()  [unwired: 2 in, 2 out]
            n122 = property on="WF-OA-002-REF" class="DigNum (strict)"("DisabledEnum"=w434) -> ()  [unwired: 2 in, 2 out]
            n123 = property on="TORQUE-REF" class="DigNum (strict)"("DisabledEnum"=w435) -> ()  [unwired: 2 in, 2 out]
            n124 = local write "NG_CL_outer_lambda"(FALSE ("NG_CL_outer_lambda")) -> ()
            n125 = local write "NG_CL_outer_IMEP"(TRUE ("NG_CL_outer_IMEP")) -> ()
            n126 = local write "NG_CL_outer_Nm"(FALSE ("NG_CL_outer_Nm")) -> ()
            n127 = local write "NG_CL_inner"(TRUE ("NG_CL_inner")) -> ()
          }
          frame 6 {
            w443 = T2."Enabled" ("Disabled")
            w442 = T2."Disabled and Grayed Out" ("Disabled")
            w441 = T2."Disabled and Grayed Out" ("Disabled")
            n128 = property on="NG_CL_outer_IMEP" class="Bool"("DisabledEnum"=w441) -> ()  [unwired: 2 in, 2 out]
            n129 = property on="NG_CL_outer_Nm" class="Bool"("DisabledEnum"=w443) -> ()  [unwired: 2 in, 2 out]
            n130 = property on="NG_CL_outer_lambda" class="Bool"("DisabledEnum"=w442) -> ()  [unwired: 2 in, 2 out]
            n131 = property on="NG-FC-001-REF" class="DigNum (strict)"("DisabledEnum"=T2."Disabled and Grayed Out" ("Disabled")) -> ()  [unwired: 2 in, 2 out]
            n132 = property on="IMEP-REF" class="DigNum (strict)"("DisabledEnum"=w441) -> ()  [unwired: 2 in, 2 out]
            n133 = property on="WF-OA-002-REF" class="DigNum (strict)"("DisabledEnum"=w442) -> ()  [unwired: 2 in, 2 out]
            n134 = property on="TORQUE-REF" class="DigNum (strict)"("DisabledEnum"=w443) -> ()  [unwired: 2 in, 2 out]
            n135 = local write "NG_CL_outer_lambda"(FALSE ("NG_CL_outer_lambda")) -> ()
            n136 = local write "NG_CL_outer_IMEP"(FALSE ("NG_CL_outer_IMEP")) -> ()
            n137 = local write "NG_CL_outer_Nm"(TRUE ("NG_CL_outer_Nm")) -> ()
            n138 = local write "NG_CL_inner"(TRUE ("NG_CL_inner")) -> ()
          }
        }
        n139 = Multiply(x=w122, y=w123) -> (x*y=w124:i16)
        n140 = Add(x=w132, y=w131) -> (x+y=w126:i16)
        "Toil control mode" <- w126
        n141 = Subtract(x=i16 2, y=w159) -> (x-y=w154:i16)
        "FV301_Ctrl_Mode" <- w154
        n142 = Subtract(x=i16 2, y=w168) -> (x-y=w156:i16)
        "PV103_Ctrl_Mode" <- w156
        n143 = Add(x=w139, y=w138) -> (x+y=w136:i16)
        "Texh control mode" <- w136
        n144 = Add(x=w118, y=w117) -> (x+y=w114:i16)
        "O2 control mode" <- w114
        n145 = Add(x=w109, y=w108) -> (x+y=w103:i16)
        "Ar control mode" <- w103
        n146 = Add(x=w124, y=w123) -> (x+y=w120:i16)
        "Tcoolant control  mode" <- w120
        n147 = Build Array(w156, w155, w154) -> (w153:i16[])
        n148 = local write "Send2MTRuint16"(w153) -> ()
        n149 = local write "TORQUE-REF"(w223) -> ()
        n150 = Greater Than 0?(x=w149) -> (x > 0?=w148:bool)
        "OverrideFromMain" <- w148
        n151 = local write "WF-OA-002-REF"(w225) -> ()
        n152 = local write "IMEP-REF"(w224) -> ()
        n153 = case shown="3" w103 {
          frame 0, Default {
            n154 = property on="WF-PT-003-REF" class="DigNum (strict)"("DisabledEnum"=T2."Disabled and Grayed Out" ("Disabled")) -> ()  [unwired: 2 in, 2 out]
            n155 = property on="AR-FT-001-REF" class="DigNum (strict)"("DisabledEnum"=T2."Disabled and Grayed Out" ("Disabled")) -> ()  [unwired: 2 in, 2 out]
            n156 = property on="AR-PC-002-REF" class="DigNum (strict)"("DisabledEnum"=T2."Disabled and Grayed Out" ("Disabled")) -> ()  [unwired: 2 in, 2 out]
          }
          frame 3 {
            n157 = local read "OverrideFromMain"() -> (w400:bool)
            n158 = Select(t=T2."Disabled and Grayed Out" ("Disabled"), s=w400, f=T2."Enabled" ("Disabled")) -> (s? t:f=w398:T2)
            n159 = property on="WF-PT-003-REF" class="DigNum (strict)"("DisabledEnum"=w398) -> ()  [unwired: 2 in, 2 out]
            n160 = property on="AR-PC-002-REF" class="DigNum (strict)"("DisabledEnum"=T2."Disabled and Grayed Out" ("Disabled")) -> ()  [unwired: 2 in, 2 out]
            n161 = property on="AR-FT-001-REF" class="DigNum (strict)"("DisabledEnum"=T2."Disabled and Grayed Out" ("Disabled")) -> ()  [unwired: 2 in, 2 out]
          }
          frame 2 {
            n162 = property on="WF-PT-003-REF" class="DigNum (strict)"("DisabledEnum"=T2."Disabled and Grayed Out" ("Disabled")) -> ()  [unwired: 2 in, 2 out]
            n163 = property on="AR-FT-001-REF" class="DigNum (strict)"("DisabledEnum"=T2."Enabled" ("Disabled")) -> ()  [unwired: 2 in, 2 out]
            n164 = property on="AR-PC-002-REF" class="DigNum (strict)"("DisabledEnum"=T2."Disabled and Grayed Out" ("Disabled")) -> ()  [unwired: 2 in, 2 out]
          }
          frame 1 {
            n165 = property on="WF-PT-003-REF" class="DigNum (strict)"("DisabledEnum"=T2."Disabled and Grayed Out" ("Disabled")) -> ()  [unwired: 2 in, 2 out]
            n166 = property on="AR-FT-001-REF" class="DigNum (strict)"("DisabledEnum"=T2."Disabled and Grayed Out" ("Disabled")) -> ()  [unwired: 2 in, 2 out]
            n167 = property on="AR-PC-002-REF" class="DigNum (strict)"("DisabledEnum"=T2."Enabled" ("Disabled")) -> ()  [unwired: 2 in, 2 out]
          }
        }
        n168 = case shown="True" w148 {
          tunnel: w147 -> [_ w331]
          tunnel: w146 -> [_ w330]
          tunnel: w145 -> [_ w332]
          frame False {
          }
          frame True {
            n169 = local write "WF-PT-003-REF"(w331) -> ()
            n170 = local write "WF-OA-001-REF"(w330) -> ()
            n171 = local write "AIC201_CO2_ConcTarget"(w332) -> ()
          }
        }
        n172 = case shown="2" w114 {
          frame 1 {
            n173 = property on="O2-FC-001-REF" class="DigNum (strict)"("DisabledEnum"=T2."Enabled" ("Disabled")) -> ()  [unwired: 2 in, 2 out]
            n174 = property on="WF-OA-001-REF" class="DigNum (strict)"("DisabledEnum"=T2."Disabled and Grayed Out" ("Disabled")) -> ()  [unwired: 2 in, 2 out]
          }
          frame 0, Default {
            n175 = property on="O2-FC-001-REF" class="DigNum (strict)"("DisabledEnum"=T2."Disabled and Grayed Out" ("Disabled")) -> ()  [unwired: 2 in, 2 out]
            n176 = property on="WF-OA-001-REF" class="DigNum (strict)"("DisabledEnum"=T2."Disabled and Grayed Out" ("Disabled")) -> ()  [unwired: 2 in, 2 out]
          }
          frame 2 {
            n177 = local read "OverrideFromMain"() -> (w390:bool)
            n178 = Select(t=T2."Disabled and Grayed Out" ("Disabled"), s=w390, f=T2."Enabled" ("Disabled")) -> (s? t:f=w389:T2)
            n179 = property on="WF-OA-001-REF" class="DigNum (strict)"("DisabledEnum"=w389) -> ()  [unwired: 2 in, 2 out]
            n180 = property on="O2-FC-001-REF" class="DigNum (strict)"("DisabledEnum"=T2."Disabled and Grayed Out" ("Disabled")) -> ()  [unwired: 2 in, 2 out]
          }
        }
        n181 = case shown="0, Default" w120 {
          frame 2 {
            n182 = property on="EC-FC-001-REF" class="DigNum (strict)"("DisabledEnum"=T2."Disabled and Grayed Out" ("Disabled")) -> ()  [unwired: 2 in, 2 out]
            n183 = property on="EC-TT-001-REF" class="DigNum (strict)"("DisabledEnum"=T2."Enabled" ("Disabled")) -> ()  [unwired: 2 in, 2 out]
          }
          frame 1 {
            n184 = property on="EC-FC-001-REF" class="DigNum (strict)"("DisabledEnum"=T2."Enabled" ("Disabled")) -> ()  [unwired: 2 in, 2 out]
            n185 = property on="EC-TT-001-REF" class="DigNum (strict)"("DisabledEnum"=T2."Disabled and Grayed Out" ("Disabled")) -> ()  [unwired: 2 in, 2 out]
          }
          frame 0, Default {
            n186 = property on="EC-FC-001-REF" class="DigNum (strict)"("DisabledEnum"=T2."Disabled and Grayed Out" ("Disabled")) -> ()  [unwired: 2 in, 2 out]
            n187 = property on="EC-TT-001-REF" class="DigNum (strict)"("DisabledEnum"=T2."Disabled and Grayed Out" ("Disabled")) -> ()  [unwired: 2 in, 2 out]
          }
        }
        n188 = case shown="3" w136 {
          frame 1 {
            n189 = property on="SW-FT-002-REF" class="DigNum (strict)"("DisabledEnum"=T2."Disabled and Grayed Out" ("Disabled")) -> ()  [unwired: 2 in, 2 out]
            n190 = property on="WF-TT-004-REF" class="DigNum (strict)"("DisabledEnum"=T2."Disabled and Grayed Out" ("Disabled")) -> ()  [unwired: 2 in, 2 out]
            n191 = property on="SW-FC-004-REF" class="DigNum (strict)"("DisabledEnum"=T2."Enabled" ("Disabled")) -> ()  [unwired: 2 in, 2 out]
          }
          frame 0, Default {
            n192 = property on="SW-FT-002-REF" class="DigNum (strict)"("DisabledEnum"=T2."Disabled and Grayed Out" ("Disabled")) -> ()  [unwired: 2 in, 2 out]
            n193 = property on="WF-TT-004-REF" class="DigNum (strict)"("DisabledEnum"=T2."Disabled and Grayed Out" ("Disabled")) -> ()  [unwired: 2 in, 2 out]
            n194 = property on="SW-FC-004-REF" class="DigNum (strict)"("DisabledEnum"=T2."Disabled and Grayed Out" ("Disabled")) -> ()  [unwired: 2 in, 2 out]
          }
          frame 2 {
            n195 = property on="SW-FT-002-REF" class="DigNum (strict)"("DisabledEnum"=T2."Enabled" ("Disabled")) -> ()  [unwired: 2 in, 2 out]
            n196 = property on="WF-TT-004-REF" class="DigNum (strict)"("DisabledEnum"=T2."Disabled and Grayed Out" ("Disabled")) -> ()  [unwired: 2 in, 2 out]
            n197 = property on="SW-FC-004-REF" class="DigNum (strict)"("DisabledEnum"=T2."Disabled and Grayed Out" ("Disabled")) -> ()  [unwired: 2 in, 2 out]
          }
          frame 3 {
            n198 = property on="SW-FT-002-REF" class="DigNum (strict)"("DisabledEnum"=T2."Disabled and Grayed Out" ("Disabled")) -> ()  [unwired: 2 in, 2 out]
            n199 = property on="WF-TT-004-REF" class="DigNum (strict)"("DisabledEnum"=T2."Enabled" ("Disabled")) -> ()  [unwired: 2 in, 2 out]
            n200 = property on="SW-FC-004-REF" class="DigNum (strict)"("DisabledEnum"=T2."Disabled and Grayed Out" ("Disabled")) -> ()  [unwired: 2 in, 2 out]
          }
        }
        n201 = case shown="False" "MTR_BackPressure_CL" {
          frame True {
            n202 = property on="PV300_VlvPosTarget_pc" class="DigNum (strict)"("DisabledEnum"=T2."Disabled and Grayed Out" ("Disabled")) -> ()  [unwired: 2 in, 2 out]
            n203 = property on="PV300_PressTarget_kPa" class="DigNum (strict)"("DisabledEnum"=T2."Enabled" ("Disabled")) -> ()  [unwired: 2 in, 2 out]
          }
          frame False, Default {
            n204 = property on="PV300_VlvPosTarget_pc" class="DigNum (strict)"("DisabledEnum"=T2."Enabled" ("Disabled")) -> ()  [unwired: 2 in, 2 out]
            n205 = property on="PV300_PressTarget_kPa" class="DigNum (strict)"("DisabledEnum"=T2."Disabled and Grayed Out" ("Disabled")) -> ()  [unwired: 2 in, 2 out]
          }
        }
        n206 = case shown="0, Default" w168 {
          frame 0, Default {
            n207 = property on="PV103_VlvPosTarget_pc" class="DigNum (strict)"("DisabledEnum"=T2."Enabled" ("Disabled")) -> ()  [unwired: 2 in, 2 out]
            n208 = property on="PV103_PressTarget_kPa" class="DigNum (strict)"("DisabledEnum"=T2."Disabled and Grayed Out" ("Disabled")) -> ()  [unwired: 2 in, 2 out]
            n209 = property on="AIC103_CO2_ConcTarget" class="DigNum (strict)"("DisabledEnum"=T2."Disabled and Grayed Out" ("Disabled")) -> ()  [unwired: 2 in, 2 out]
          }
          frame 1 {
            n210 = property on="PV103_VlvPosTarget_pc" class="DigNum (strict)"("DisabledEnum"=T2."Disabled and Grayed Out" ("Disabled")) -> ()  [unwired: 2 in, 2 out]
            n211 = property on="PV103_PressTarget_kPa" class="DigNum (strict)"("DisabledEnum"=T2."Enabled" ("Disabled")) -> ()  [unwired: 2 in, 2 out]
            n212 = property on="AIC103_CO2_ConcTarget" class="DigNum (strict)"("DisabledEnum"=T2."Disabled and Grayed Out" ("Disabled")) -> ()  [unwired: 2 in, 2 out]
          }
          frame 2 {
            n213 = property on="PV103_VlvPosTarget_pc" class="DigNum (strict)"("DisabledEnum"=T2."Disabled and Grayed Out" ("Disabled")) -> ()  [unwired: 2 in, 2 out]
            n214 = property on="PV103_PressTarget_kPa" class="DigNum (strict)"("DisabledEnum"=T2."Disabled and Grayed Out" ("Disabled")) -> ()  [unwired: 2 in, 2 out]
            n215 = property on="AIC103_CO2_ConcTarget" class="DigNum (strict)"("DisabledEnum"=T2."Enabled" ("Disabled")) -> ()  [unwired: 2 in, 2 out]
          }
        }
        n216 = case shown="0, Default" w126 {
          frame 1 {
            n217 = property on="SW-FC-008-REF" class="DigNum (strict)"("DisabledEnum"=T2."Enabled" ("Disabled")) -> ()  [unwired: 2 in, 2 out]
            n218 = property on="SW-FT-004-REF" class="DigNum (strict)"("DisabledEnum"=T2."Disabled and Grayed Out" ("Disabled")) -> ()  [unwired: 2 in, 2 out]
            n219 = property on="EO-TT-001-REF" class="DigNum (strict)"("DisabledEnum"=T2."Disabled and Grayed Out" ("Disabled")) -> ()  [unwired: 2 in, 2 out]
          }
          frame 0, Default {
            n220 = property on="SW-FC-008-REF" class="DigNum (strict)"("DisabledEnum"=T2."Disabled and Grayed Out" ("Disabled")) -> ()  [unwired: 2 in, 2 out]
            n221 = property on="SW-FT-004-REF" class="DigNum (strict)"("DisabledEnum"=T2."Disabled and Grayed Out" ("Disabled")) -> ()  [unwired: 2 in, 2 out]
            n222 = property on="EO-TT-001-REF" class="DigNum (strict)"("DisabledEnum"=T2."Disabled and Grayed Out" ("Disabled")) -> ()  [unwired: 2 in, 2 out]
          }
          frame 2 {
            n223 = property on="SW-FC-008-REF" class="DigNum (strict)"("DisabledEnum"=T2."Disabled and Grayed Out" ("Disabled")) -> ()  [unwired: 2 in, 2 out]
            n224 = property on="SW-FT-004-REF" class="DigNum (strict)"("DisabledEnum"=T2."Enabled" ("Disabled")) -> ()  [unwired: 2 in, 2 out]
            n225 = property on="EO-TT-001-REF" class="DigNum (strict)"("DisabledEnum"=T2."Disabled and Grayed Out" ("Disabled")) -> ()  [unwired: 2 in, 2 out]
          }
          frame 3 {
            n226 = property on="SW-FC-008-REF" class="DigNum (strict)"("DisabledEnum"=T2."Disabled and Grayed Out" ("Disabled")) -> ()  [unwired: 2 in, 2 out]
            n227 = property on="SW-FT-004-REF" class="DigNum (strict)"("DisabledEnum"=T2."Disabled and Grayed Out" ("Disabled")) -> ()  [unwired: 2 in, 2 out]
            n228 = property on="EO-TT-001-REF" class="DigNum (strict)"("DisabledEnum"=T2."Enabled" ("Disabled")) -> ()  [unwired: 2 in, 2 out]
          }
        }
        n229 = case shown="0, Default" w159 {
          frame 0, Default {
            n230 = property on="FV301_VlvPosTarget_pc" class="DigNum (strict)"("DisabledEnum"=T2."Enabled" ("Disabled")) -> ()  [unwired: 2 in, 2 out]
            n231 = property on="FV301_FlowTarget_kgh" class="DigNum (strict)"("DisabledEnum"=T2."Disabled and Grayed Out" ("Disabled")) -> ()  [unwired: 2 in, 2 out]
            n232 = property on="AIC201_CO2_ConcTarget" class="DigNum (strict)"("DisabledEnum"=T2."Disabled and Grayed Out" ("Disabled")) -> ()  [unwired: 2 in, 2 out]
          }
          frame 1 {
            n233 = property on="FV301_VlvPosTarget_pc" class="DigNum (strict)"("DisabledEnum"=T2."Disabled and Grayed Out" ("Disabled")) -> ()  [unwired: 2 in, 2 out]
            n234 = property on="FV301_FlowTarget_kgh" class="DigNum (strict)"("DisabledEnum"=T2."Enabled" ("Disabled")) -> ()  [unwired: 2 in, 2 out]
            n235 = property on="AIC201_CO2_ConcTarget" class="DigNum (strict)"("DisabledEnum"=T2."Disabled and Grayed Out" ("Disabled")) -> ()  [unwired: 2 in, 2 out]
          }
          frame 2 {
            n236 = property on="FV301_VlvPosTarget_pc" class="DigNum (strict)"("DisabledEnum"=T2."Disabled and Grayed Out" ("Disabled")) -> ()  [unwired: 2 in, 2 out]
            n237 = property on="FV301_FlowTarget_kgh" class="DigNum (strict)"("DisabledEnum"=T2."Disabled and Grayed Out" ("Disabled")) -> ()  [unwired: 2 in, 2 out]
            n238 = property on="AIC201_CO2_ConcTarget" class="DigNum (strict)"("DisabledEnum"=T2."Enabled" ("Disabled")) -> ()  [unwired: 2 in, 2 out]
          }
        }
        n239 = local read "NG_CL_inner"() -> (w212:bool)
        n240 = Select(t=w215, s=w212, f=0.0 ("NG-FC-001-REF")) -> (s? t:f=w213:dbl)
        n241 = local write "NG-FC-001-REF"(w213) -> ()
      }
      n242 = while {
        stop <- FALSE ("Modbus STOP") stop-if-true
        n243 = flat-sequence {
          frame #0 {
            (unwired) "localhost" ("address")
            n244 = call-poly <vilib>:"Create Master Instance.vi"("port (502)"="port (502)", "address"="Slave address") -> ("error out"=w11:errorcluster, "TCP master instance"=w12:refnum<class "Modbus Master.lvclass">)  [unwired: 8 in]
            n245 = while {
              shift-right: [w61] -> w15
              shift-left: w11 -> [w51]
              shift-right: [w71] -> w14
              shift-left: w12 -> [w52]
              stop <- w73 stop-if-true
              # "Read Operation"
              n246 = Wait (ms)(milliseconds to wait=u32 1000) -> ()  [unwired: 1 out]
              n247 = call "APC_9049_float2u16.vi"("min"="min", "holding register values"="Send2MTRfloats", "max"="max") -> ("uint16 array"=w58:u16[])
              n248 = call-dynamic "Read Holding Registers.vi"("error in (no error)"=w51, "number of holding registers"=u16 7, "starting address"=u16 40001, "Modbus master in"=w52) -> ("error out"=w68:errorcluster, "register values"=w36:u16[], "Modbus master out"=w71:refnum<class "Modbus Master.lvclass">)  [unwired: 5 in]
              "MTR modbus u16" <- w36
              n249 = call-dynamic "Read Holding Registers.vi"("error in (no error)"=w68, "number of holding registers"=u16 38, "starting address"=u16 41001, "Modbus master in"=w52) -> ("error out"=w65:errorcluster, "register values"=w55:u16[])  [unwired: 5 in, 1 out]
              n250 = call-dynamic "Write Multiple Holding Registers.vi"("error in (no error)"=w65, "holding register values"="Send2MTRuint16", "starting address"=u16 45001, "Modbus master in"=w52) -> ("error out"=w64:errorcluster)  [unwired: 6 in, 1 out]
              n251 = call-dynamic "Write Multiple Holding Registers.vi"("error in (no error)"=w64, "holding register values"=w58, "starting address"=u16 46001, "Modbus master in"=w52) -> ("error out"=w61:errorcluster)  [unwired: 6 in, 1 out]
              "error out" <- w61
              n252 = call "APC_9049_u162float.vi"("min"="min 2", "holding register values"=w55, "max"="max 2") -> ("Array"=w50:sgl[])
              "MTR modbus floats" <- w50
              n253 = Index Array(array=w36, index #1=0 ("index")) -> (element #1=w35:u16, element #2=w24:u16, element #3=w33:u16, element #7=w29:u16)  [unwired: 6 in, 3 out]
              n254 = Equal To 0?(x=w35) -> (x = 0?=→"Control from LV":bool)
              n255 = Index Array(array=w50, index #1=0 ("index")) -> (element #2=w48:sgl, element #4=w47:sgl, element #6=w46:sgl, element #8=w45:sgl, element #10=w44:sgl, element #12=w43:sgl, element #14=w42:sgl, element #16=w41:sgl, element #17=w40:sgl, element #18=w39:sgl, element #19=w38:sgl)  [unwired: 18 in, 8 out]
              n256 = Number To Boolean Array(number=w29) -> (Boolean array=→"MTR errors":bool[])
              n257 = Quotient & Remainder(x=w33, y=u16 2) -> (x-y*floor(x/y)=w31:u16)  [unwired: 1 out]
              n258 = local write "FT301_Flow_kgh"(w44) -> ()
              n259 = local write "AT103_CO2Conc"(w48) -> ()
              n260 = local write "PT103_Pressure_kPa"(w47) -> ()
              n261 = local write "PV103_VlvPos_pc_fb"(w46) -> ()
              n262 = local write "AT201_CO2Conc"(w45) -> ()
              n263 = local write "FV301_VlvPos_pc_fb"(w43) -> ()
              n264 = local write "PT300_Pressure_kPa"(w42) -> ()
              n265 = local write "PV300_VlvPos_pc_fb"(w41) -> ()
              n266 = local write "C101_CompSpeed_rpm"(w40) -> ()
              n267 = local write "PT104_Pressure_kPa"(w39) -> ()
              n268 = local write "PT106_Pressure_kPa"(w38) -> ()
              n269 = Equal To 0?(x=w31) -> (x = 0?=→"HB":bool)
              n270 = Decrement(x=w24) -> (x-1=w25:u16)
              n271 = Replace Array Subset(array=bool[] [FALSE, FALSE, FALSE, FALSE, FALSE, FALSE, FALSE], new element=TRUE ("new element/subarray"), index=w25) -> (w22:bool[])
              n272 = Or(x=w61, y=FALSE ("Modbus STOP")) -> (x .or. y?=w73:bool)
              n273 = Index Array(array=w22, index #1=0 ("index")) -> (element #1=→"Idle":bool, element #2=→"Start":bool, element #3=→"Pre-operation":bool, element #4=→"Operation":bool, element #5=→"Shutdown":bool, element #6=→"Emergency shutdown":bool)  [unwired: 5 in]
            }
            n274 = call-dynamic "Close.vi"("error in (no error)"=w15, "Modbus master in"=w14) -> ()  [unwired: 9 in, 1 out]
          }
          frame #1 {
            # "if communication is lost, wait and retry"
            n275 = Wait (ms)(milliseconds to wait=u32 5000) -> ()  [unwired: 1 out]
          }
        }
      }
      n276 = while {
        stop <- FALSE stop-if-true
        n277 = case shown="True" "Clear warning" {
          frame False {
          }
          frame True {
            n278 = local write "Clear warning"(FALSE ("Clear warning request")) -> ()
            n279 = call "APC_ClearErrorButton.vi"() -> ()  [unwired: 1 in]
          }
        }
        n280 = Wait Until Next ms Multiple(millisecond multiple=u32 200) -> ()  [unwired: 1 out]
      }
    }
    frame #1 {
      (unwired) FALSE ("EMERGENCY STOP")
    }
  }
